vi "fgt set sensor Regulation Response.vi"(8 "error in (no error)":errorcluster, 10 "responseTime":u32, 11 "sensorIndex":u32) -> (0 "error out":errorcluster)   [LabVIEW 2020, in "fgt_SDK.lvlib"]
doc: "Set on a running regulation pressure response time. Minimal value is 2 for FlowEZ, 6 for MFCS controllers.\nThis function is useful if a more smooth response is wanted. Not supported by IPS."
uses:
  fgt_SDK.lvlib
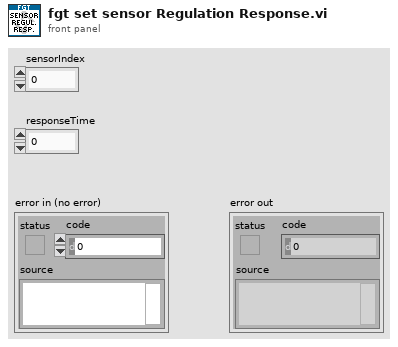
[diagram p1: front panel]
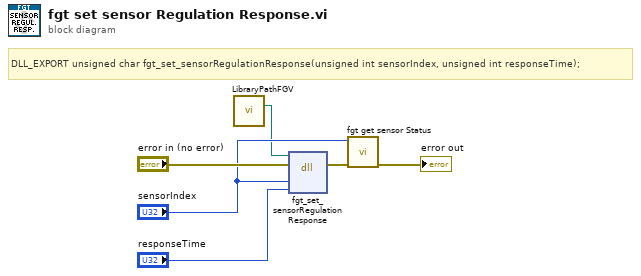
[diagram p0: block diagram]
diagram:
  # "DLL_EXPORT unsigned char fgt_set_sensorRegulationResponse(unsigned int sensorIndex, unsigned int responseTime);"
  n1 = call "LibraryPathFGV.vi"() -> ("Path Out"=w1:path)  [unwired: 14 in, 1 out]
  n2 = dll-call lib="C:/Workspace/fgt-SDK/LabVIEW/dlls/fgt_SDK_*.*" fn="fgt_set_sensorRegulationResponse"(path in=w1, error in="error in (no error)", "sensorIndex"="sensorIndex", "responseTime"="responseTime") -> (error out=w4:errorcluster)  [unwired: 4 in, 1 out]
  n3 = call "fgt get sensor Status.vi"("error in (no error)"=w4, "pressureIndex"="sensorIndex") -> ("error out"=→"error out":errorcluster)  [unwired: 9 in]
